vi "CRYCursor Show.vi"(6 "Flattened Cursor Property":string, 11 "pGraph VI":refnum<vi>) -> ()   [LabVIEW 2013]
uses:
  Control/CRYCursor Property.ctl
panel:
  in  "Cursor Property":T1[](array[typedef])
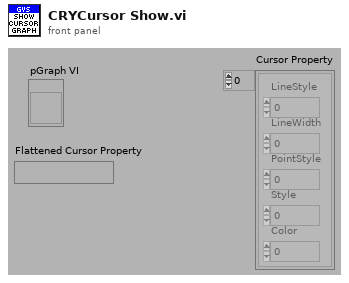
[diagram p1: front panel]
types:
  T1 = typedef "CRYCursor Property.ctl" = cluster{"LineStyle":u8, "LineWidth":u8, "PointStyle":u8, "Style":u8, "Color":u32}
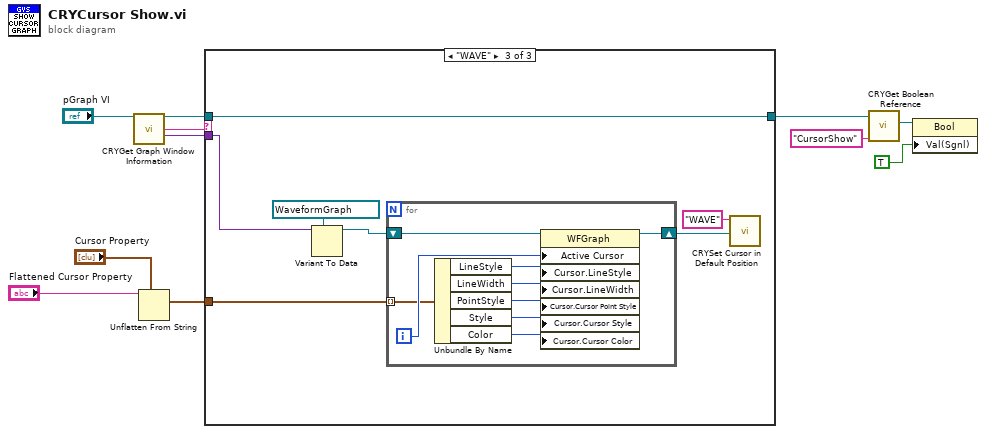
[diagram p0: block diagram]
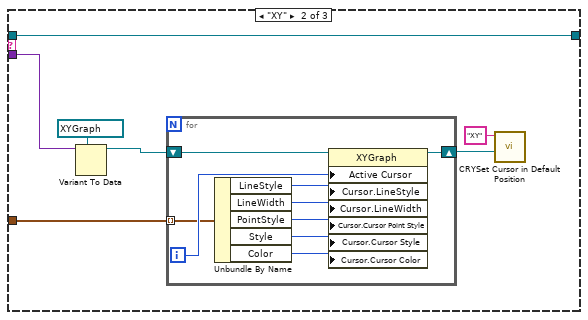
[diagram p3: hidden frame]
diagram:
  n1 = call "CRYGet Graph Window Information.vi"("pGraph VI In"="pGraph VI") -> ("pGraph VI Out"=w1:refnum<vi>, "Graph Type Out"=w3:string, "Graph Control Ref Out"=w4:variant)  [unwired: 4 in, 8 out]
  n2 = Unflatten From String(type="Cursor Property", binary string="Flattened Cursor Property") -> (value=w6:T1[])  [unwired: 3 in, 2 out]
  n3 = case shown="\"WAVE\"" w3 {
    tunnel: w4 -> [_ w19 w35]
    tunnel: w6 -> [_ w17 w34]
    tunnel: [w12 w16 w32] -> w5
    tunnel: w1 -> [w12 w16 w32]
    frame Default {
    }
    frame "XY" {
      n4 = Variant To Data(type=refnum<vi> refnum ("XY Graph"), Variant=w19) -> (data=w15:refnum<vi>)  [unwired: 1 in, 1 out]
      n5 = for {
        tunnel: w17 -> [w27] mode=indexing
        shift-right: [w20] -> w13
        shift-left: w15 -> [w21]
        i -> [w28]
        n6 = Unbundle By Name(w27) -> ("LineStyle"=w26:u8, "LineWidth"=w25:u8, "PointStyle"=w24:u8, "Style"=w23:u8, "Color"=w22:u32)
        n7 = property class="XYGraph"(reference=w21, "Active Cursor"=w28, "Cursor.LineStyle"=w26, "Cursor.LineWidth"=w25, "Cursor.Cursor Point Style"=w24, "Cursor.Cursor Style"=w23, "Cursor.Cursor Color"=w22) -> (reference out=w20:refnum<vi>)  [unwired: 1 in, 1 out]
      }
      n8 = call "CRYSet Cursor in Default Position.vi"("XY Graph Ref"=w13, "Graph Type"="XY") -> ()  [unwired: 10 in]
    }
    frame "WAVE" {
      n9 = Variant To Data(type=refnum<vi> refnum ("WaveGraph Ref"), Variant=w35) -> (data=w31:refnum<vi>)  [unwired: 1 in, 1 out]
      n10 = for {
        tunnel: w34 -> [w43] mode=indexing
        shift-right: [w36] -> w29
        shift-left: w31 -> [w37]
        i -> [w44]
        n11 = Unbundle By Name(w43) -> ("LineStyle"=w42:u8, "LineWidth"=w41:u8, "PointStyle"=w40:u8, "Style"=w39:u8, "Color"=w38:u32)
        n12 = property class="WFGraph"(reference=w37, "Active Cursor"=w44, "Cursor.LineStyle"=w42, "Cursor.LineWidth"=w41, "Cursor.Cursor Point Style"=w40, "Cursor.Cursor Style"=w39, "Cursor.Cursor Color"=w38) -> (reference out=w36:refnum<vi>)  [unwired: 1 in, 1 out]
      }
      n13 = call "CRYSet Cursor in Default Position.vi"("Wave Graph Ref"=w29, "Graph Type"="WAVE") -> ()  [unwired: 10 in]
    }
  }
  n14 = call "CRYGet Boolean Reference.vi"("Label Name"="CursorShow", "VI Refnum"=w5) -> ("Boolean Ref"=w10:refnum<vi>)  [unwired: 7 in, 2 out]
  n15 = property class="Bool"(reference=w10, "Val(Sgnl)"=TRUE ("Visible")) -> ()  [unwired: 1 in, 2 out]
